vi "VisionMain_29.vi"(7 "error in":errorcluster, 10 "Image In":T1) -> (0 "error out":errorcluster, 1 "Centroid (Centroid 1)":cluster{"X Centroid":sgl, "Y Centroid":sgl} {"Y Centroid" format="%.2f"; "X Centroid" format="%.2f"}, 2 "Particle Measurements (Pixels) (Particle Analysis 1)":dbl[][](array[numeric]) format="%.2f", 3 "Image Out":T1, 4 "Number of Particles (Particle Analysis 1)":i32)   [LabVIEW 2016]
uses:
  <vilib>/vision/Image Controls.llb/IMAQ Image.ctl
  <vilib>/vision/NI_Vision_Development_Module.lvlib
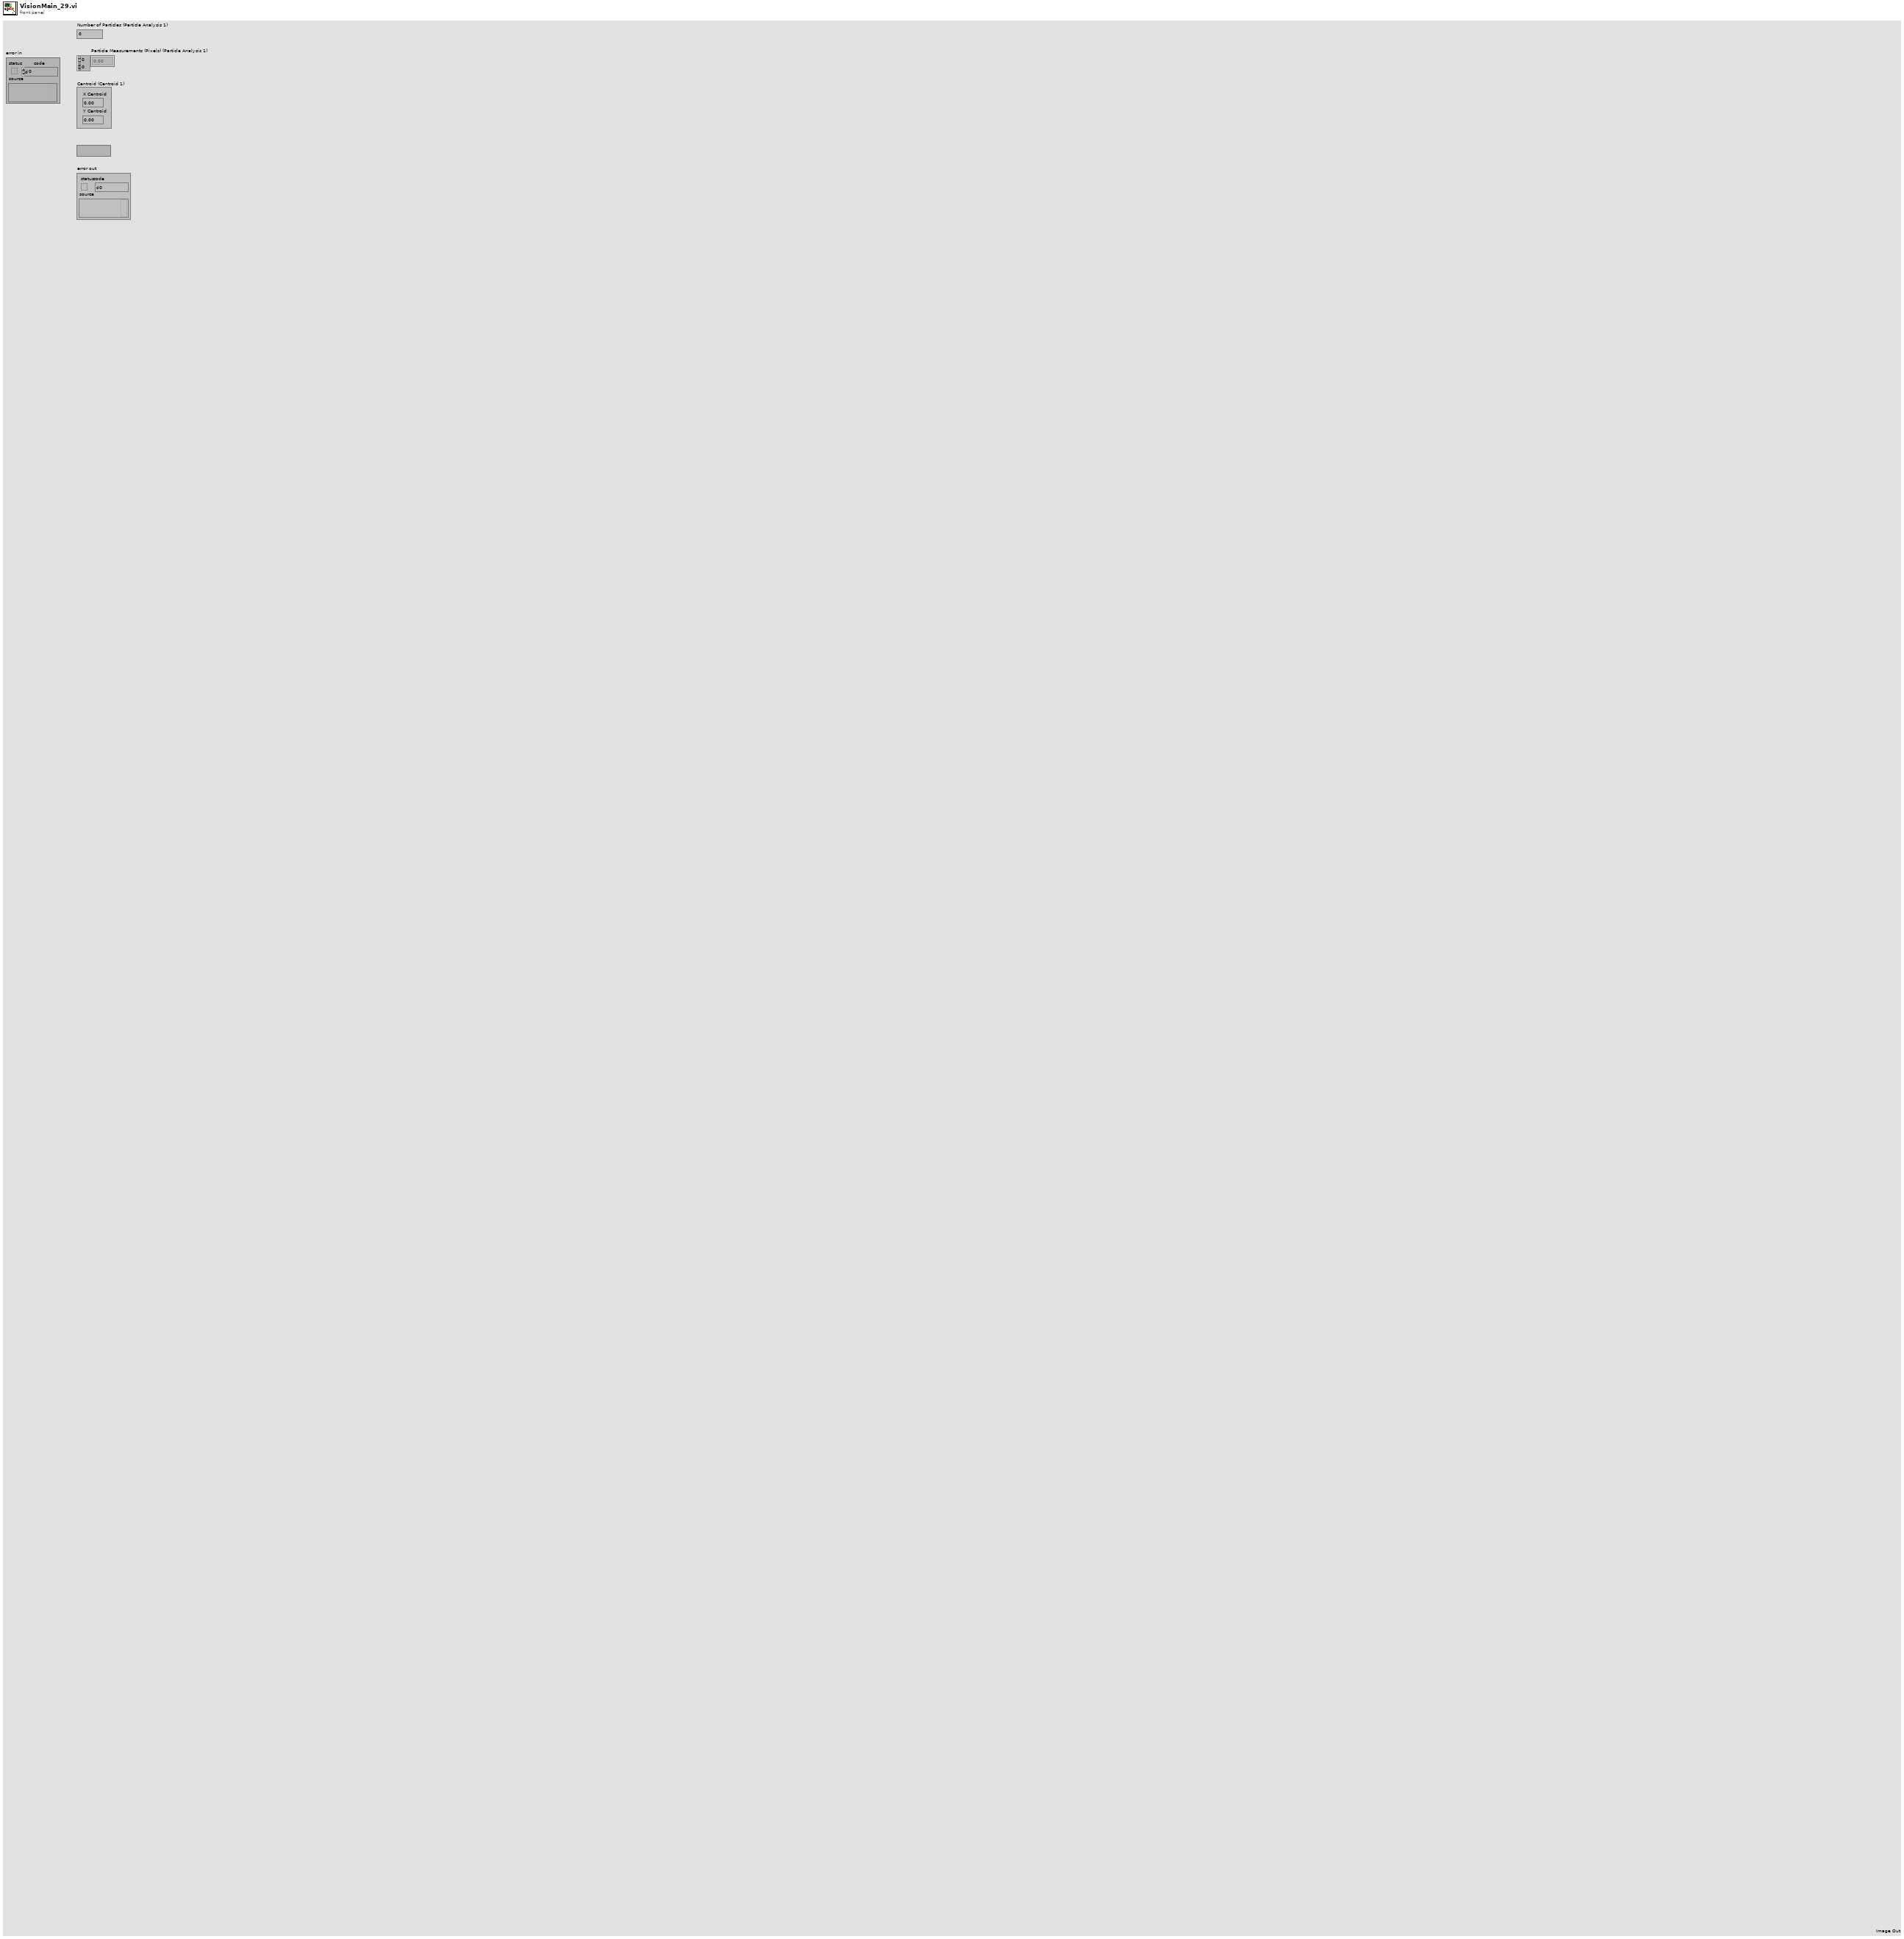
[diagram p1: front panel]
types:
  T1 = typedef "IMAQ Image.ctl" = refnum<image>
  T2 = cluster{"Measurement Parameter":i32, "Range Lower Value":dbl, "Range Upper Value":dbl, "Range":bool, "Measurement Type":bool}[]
  T3 = cluster{"Brightness":sgl, "Contrast":sgl, "Gamma":sgl}
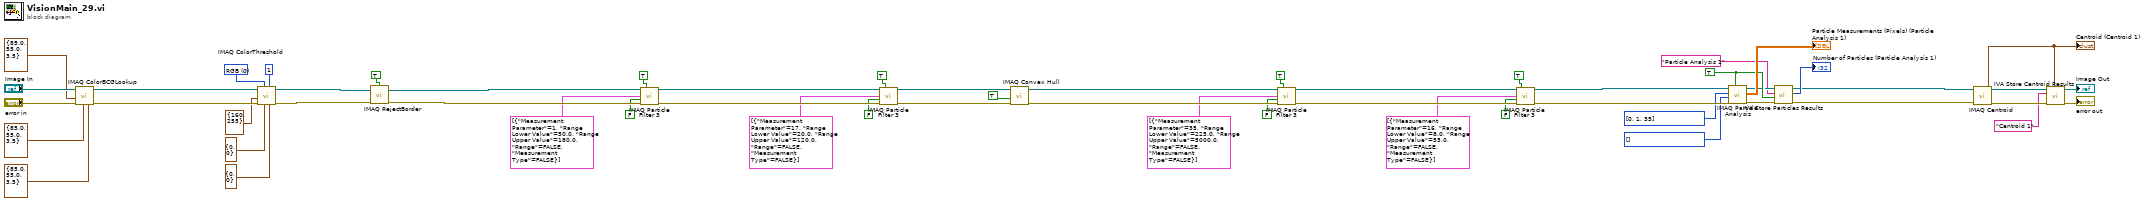
[diagram p0: block diagram]
diagram:
  w15 = i32[] [] items=["Center of Mass X", "Center of Mass Y", "First Pixel X", "First Pixel Y", "Bounding Rect Left", "Bounding Rect Top", "Bounding Rect Right", "Bounding Rect Bottom", "Max Feret Diameter Start X", "Max Feret Diameter Start Y", "Max Feret Diameter End X", "Max Feret Diameter End Y", "Max Horiz. Segment Length Left", "Max Horiz. Segment Length Right", "Max Horiz. Segment Length Row", "-", "Bounding Rect Width", "Bounding Rect Height", "Bounding Rect Diagonal", "Perimeter", "Convex Hull Perimeter", "Holes' Perimeter", "Max Feret Diameter", "Equivalent Ellipse Major Axis", "Equivalent Ellipse Minor Axis", "Equivalent Ellipse Minor Axis (Feret)", "Equivalent Rect Long Side", "Equivalent Rect Short Side", "Equivalent Rect Diagonal", "Equivalent Rect Short Side (Feret)", "Average Horiz. Segment Length", "Average Vert. Segment Length", "Hydraulic Radius", "Waddel Disk Diameter", "-", "Area", "Holes' Area", "Particle & Holes' Area", "Convex Hull Area", "Image Area", "-", "Number of Holes", "Number of Horiz. Segments", "Number of Vert. Segments", "-", "Orientation", "Max Feret Diameter Orientation", "-", "% Area/Image Area", "% Area/(Particle & Holes' Area)", "Ratio of Equivalent Ellipse Axes", "Ratio of Equivalent Rect Sides", "-", "Elongation Factor", "Compactness Factor", "Heywood Circularity Factor", "Type Factor", "-", "Sum X", "Sum Y", "Sum XX", "Sum XY", "Sum YY", "Sum XXX", "Sum XXY", "Sum XYY", "Sum YYY", "-", "Moment of Inertia XX", "Moment of Inertia XY", "Moment of Inertia YY", "Moment of Inertia XXX", "Moment of Inertia XXY", "Moment of Inertia XYY", "Moment of Inertia YYY", "Norm. Moment of Inertia XX", "Norm. Moment of Inertia XY", "Norm. Moment of Inertia YY", "Norm. Moment of Inertia XXX", "Norm. Moment of Inertia XXY", "Norm. Moment of Inertia XYY", "Norm. Moment of Inertia YYY", "Hu Moment 1", "Hu Moment 2", "Hu Moment 3", "Hu Moment 4", "Hu Moment 5", "Hu Moment 6", "Hu Moment 7"] ("Real-World Measurements")
  w16 = i32[] [0, 1, 35] items=["Center of Mass X", "Center of Mass Y", "First Pixel X", "First Pixel Y", "Bounding Rect Left", "Bounding Rect Top", "Bounding Rect Right", "Bounding Rect Bottom", "Max Feret Diameter Start X", "Max Feret Diameter Start Y", "Max Feret Diameter End X", "Max Feret Diameter End Y", "Max Horiz. Segment Length Left", "Max Horiz. Segment Length Right", "Max Horiz. Segment Length Row", "-", "Bounding Rect Width", "Bounding Rect Height", "Bounding Rect Diagonal", "Perimeter", "Convex Hull Perimeter", "Holes' Perimeter", "Max Feret Diameter", "Equivalent Ellipse Major Axis", "Equivalent Ellipse Minor Axis", "Equivalent Ellipse Minor Axis (Feret)", "Equivalent Rect Long Side", "Equivalent Rect Short Side", "Equivalent Rect Diagonal", "Equivalent Rect Short Side (Feret)", "Average Horiz. Segment Length", "Average Vert. Segment Length", "Hydraulic Radius", "Waddel Disk Diameter", "-", "Area", "Holes' Area", "Particle & Holes' Area", "Convex Hull Area", "Image Area", "-", "Number of Holes", "Number of Horiz. Segments", "Number of Vert. Segments", "-", "Orientation", "Max Feret Diameter Orientation", "-", "% Area/Image Area", "% Area/(Particle & Holes' Area)", "Ratio of Equivalent Ellipse Axes", "Ratio of Equivalent Rect Sides", "-", "Elongation Factor", "Compactness Factor", "Heywood Circularity Factor", "Type Factor", "-", "Sum X", "Sum Y", "Sum XX", "Sum XY", "Sum YY", "Sum XXX", "Sum XXY", "Sum XYY", "Sum YYY", "-", "Moment of Inertia XX", "Moment of Inertia XY", "Moment of Inertia YY", "Moment of Inertia XXX", "Moment of Inertia XXY", "Moment of Inertia XYY", "Moment of Inertia YYY", "Norm. Moment of Inertia XX", "Norm. Moment of Inertia XY", "Norm. Moment of Inertia YY", "Norm. Moment of Inertia XXX", "Norm. Moment of Inertia XXY", "Norm. Moment of Inertia XYY", "Norm. Moment of Inertia YYY", "Hu Moment 1", "Hu Moment 2", "Hu Moment 3", "Hu Moment 4", "Hu Moment 5", "Hu Moment 6", "Hu Moment 7"] ("Pixel Measurements")
  w12 = TRUE ("Connectivity 4/8 (8)")
  w48 = u16 0 items=["RGB", "HSL", "HSV", "HSI"] ("Color Mode")
  n1 = call "IMAQ ColorBCGLookup"("Blue BCG Values"=T3 {"Brightness"=85.0, "Contrast"=55.0, "Gamma"=3.5}, "Green BCG Values"=T3 {"Brightness"=85.0, "Contrast"=55.0, "Gamma"=3.5}, "error in (no error)"="error in", "Red BCG Values"=T3 {"Brightness"=85.0, "Contrast"=55.0, "Gamma"=3.5}, "Image Src"="Image In") -> ("error out"=w53:errorcluster, "Image Dst Out"=w44:T1)  [unwired: 2 in, 3 out]
  n2 = call "IMAQ ColorThreshold"("Blue or Luma or Val or Inten Range"=cluster{"Lower value":i32, "Upper value":i32} {"Lower value"=0, "Upper value"=0}, "Replace Value"=1, "Green or Sat Range"=cluster{"Lower value":i32, "Upper value":i32} {"Lower value"=0, "Upper value"=0}, "Color Mode"=w48, "error in (no error)"=w53, "Red or Hue Range"=cluster{"Lower value":i32, "Upper value":i32} {"Lower value"=160, "Upper value"=255}, "Image Src"=w44) -> ("error out"=w43:errorcluster, "Image Dst Out"=w41:T1)  [unwired: 1 in, 2 out]
  n3 = call "IMAQ RejectBorder"("error in (no error)"=w43, "Image Src"=w41, "Connectivity 4/8 (8)"=TRUE) -> ("error out"=w40:errorcluster, "Image Dst Out"=w36:T1)  [unwired: 1 in, 2 out]
  n4 = call "IMAQ Particle Filter 3"("Image Src"=w36, "Connectivity 4/8 (8)"=TRUE, "Selection Values"=T2 [{"Measurement Parameter"=1, "Range Lower Value"=50.0, "Range Upper Value"=180.0, "Range"=FALSE, "Measurement Type"=FALSE}], "Keep/Remove Particles (F)"=FALSE ("Keep/Remove Particles"), "error in (no error)"=w40) -> ("Image Dst Out"=w31:T1, "error out"=w37:errorcluster)  [unwired: 4 in, 5 out]
  n5 = call "IMAQ Particle Filter 3"("Image Src"=w31, "Connectivity 4/8 (8)"=TRUE, "Selection Values"=T2 [{"Measurement Parameter"=17, "Range Lower Value"=20.0, "Range Upper Value"=120.0, "Range"=FALSE, "Measurement Type"=FALSE}], "Keep/Remove Particles (F)"=FALSE ("Keep/Remove Particles"), "error in (no error)"=w37) -> ("Image Dst Out"=w29:T1, "error out"=w32:errorcluster)  [unwired: 4 in, 5 out]
  n6 = call "IMAQ Convex Hull"("error in (no error)"=w32, "Connectivity 4/8 (8)"=TRUE, "Image Src"=w29) -> ("error out"=w27:errorcluster, "Image Dst Out"=w23:T1)  [unwired: 1 in, 6 out]
  n7 = call "IMAQ Particle Filter 3"("Image Src"=w23, "Connectivity 4/8 (8)"=TRUE, "Selection Values"=T2 [{"Measurement Parameter"=35, "Range Lower Value"=225.0, "Range Upper Value"=5000.0, "Range"=FALSE, "Measurement Type"=FALSE}], "Keep/Remove Particles (F)"=FALSE ("Keep/Remove Particles"), "error in (no error)"=w27) -> ("Image Dst Out"=w18:T1, "error out"=w24:errorcluster)  [unwired: 4 in, 5 out]
  n8 = call "IMAQ Particle Filter 3"("Image Src"=w18, "Connectivity 4/8 (8)"=TRUE, "Selection Values"=T2 [{"Measurement Parameter"=16, "Range Lower Value"=8.0, "Range Upper Value"=55.0, "Range"=FALSE, "Measurement Type"=FALSE}], "Keep/Remove Particles (F)"=FALSE ("Keep/Remove Particles"), "error in (no error)"=w24) -> ("Image Dst Out"=w13:T1, "error out"=w19:errorcluster)  [unwired: 4 in, 5 out]
  n9 = call "IMAQ Particle Analysis"("Connectivity 4/8 (8)"=w12, "error in (no error)"=w19, "Real-World Measurements"=w15, "Pixel Measurements"=w16, "Image"=w13) -> ("error out"=w9:errorcluster, "Particle Measurements (Pixels)"=→"Particle Measurements (Pixels) (Particle Analysis 1)":dbl[][], "Image Out (duplicate)"=w11:T1)  [unwired: 4 out]
  n10 = call <vilib>:"IVA Store Particles Results.vi"("error in (no error)"=w9, "Connectivity 4/8 (8)"=w12, "Step Name"="Particle Analysis 1", "Image in"=w11) -> ("error out"=w8:errorcluster, "Number of Particles"=→"Number of Particles (Particle Analysis 1)":i32, "Image dup"=w4:T1)  [unwired: 5 out]
  n11 = call "IMAQ Centroid"("error in (no error)"=w8, "Image"=w4) -> ("error out"=w6:errorcluster, "Centroid"=w1:cluster{"X Centroid":sgl, "Y Centroid":sgl})  [unwired: 1 in, 1 out]
  "Centroid (Centroid 1)" <- w1
  n12 = call <vilib>:"IVA Store Centroid Results.vi"("Centroid in"=w1, "error in (no error)"=w6, "Step Name"="Centroid 1", "Image in"=w4) -> ("error out"=→"error out":errorcluster, "Image dup"=→"Image Out":T1)  [unwired: 6 out]
